vi "clear.vi"(0 "port number set":i32) -> ()   [LabVIEW 2019]
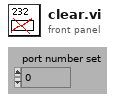
[diagram p1: front panel]
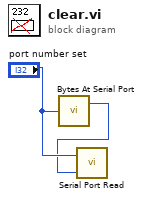
[diagram p0: block diagram]
diagram:
  n1 = call <vilib>:"Bytes At Serial Port.vi"("port number"="port number set") -> ("byte count"=w1:u32)  [unwired: 1 out]
  n2 = call <vilib>:"Serial Port Read.vi"("requested byte count"=w1, "port number"="port number set") -> ()  [unwired: 2 out]
